vi "Read Format.vi"(8 "error in (no error)":errorcluster, 11 "VISA resource name":refnum<visa-resource-name>) -> (0 "error out":errorcluster, 1 "format":i32(ring) items=["log magnitude", "phase", "delay", "Smith chart", "polar", "linear magnitude", "standing wave ratio", "real", "imaginary"], 3 "VISA resource name out":refnum<visa-resource-name>)   [LabVIEW 2018, in "Agilent 87XX Series.lvlib"]
doc: "This VI for the HP 8753B is used to read the meausurement format.\n\n0 log magnitude\n1 phase\n2 delay\n3 Smith chart\n4 polar\n5 linear magnitude\n6 standing wave ratio\n7 real\n8 imaginary"
uses:
  Agilent 87XX Series.lvlib
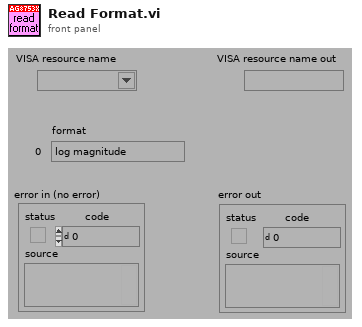
[diagram p1: front panel]
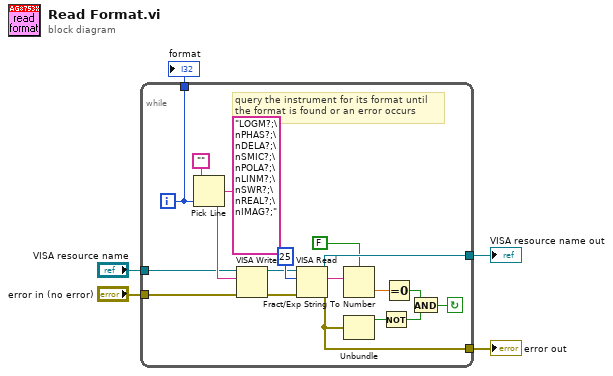
[diagram p0: block diagram]
diagram:
  n1 = while {
    tunnel: "error in (no error)" -> [w9]
    tunnel: "VISA resource name" -> [w10]
    tunnel: [w11] -> w2
    tunnel: [w12] -> w1
    tunnel: [w17] -> w5
    i -> [w17]
    stop <- w13 continue-if-true
    # "query the instrument for its format until\nthe format is found or an error occurs"
    n2 = Pick Line(string ("")="", multi-line string="LOGM?;\nPHAS?;\nDELA?;\nSMIC?;\nPOLA?;\nLINM?;\nSWR?;\nREAL?;\nIMAG?;", line index=w17) -> (output string=w21:string)
    n3 = VISA Write(VISA resource name=w10, write buffer=w21, error in (no error)=w9) -> (VISA resource name out=w7:refnum<visa-resource-name>, error out=w20:errorcluster)  [unwired: 1 out]
    n4 = VISA Read(VISA resource name=w7, byte count=u32 25, error in (no error)=w20) -> (VISA resource name out=w11:refnum<visa-resource-name>, read buffer=w19:string, error out=w12:errorcluster)  [unwired: 1 out]
    n5 = Fract/Exp String To Number(use system decimal point (T)=FALSE, string=w19) -> (number=w18:dbl)  [unwired: 2 in, 1 out]
    n6 = Unbundle(w12) -> ("status"=w16:bool)  [unwired: 2 out]
    n7 = Not(x=w16) -> (.not. x?=w14:bool)
    n8 = Equal To 0?(x=w18) -> (x = 0?=w15:bool)
    n9 = And(x=w15, y=w14) -> (x .and. y?=w13:bool)
  }
  "format" <- w5
  "VISA resource name out" <- w2
  "error out" <- w1
